vi "5492_OrientationButtonPress.vi"() -> ()   [LabVIEW 2016]
panel:
  in  "Boolean":bool
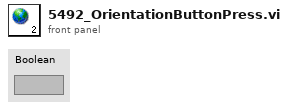
[diagram p1: front panel]
diagram:
